vi "Main.vi"() -> ()   [LabVIEW 2020]
panel:
  out "Homogenization Process":u8(slide) scale=0.0..100.0
  out "Internet Connections":string
  out "Raw Material Prices (MYR)":string[][](array[string])
  out "Event Logging":string[][](array[string])
  in  "C\nSell Stock: 3":dbl min=0.0 max=600.0 step=1.0
  in  "Sell Button C":bool
  in  "B\nSell Stock: 2":dbl=1.0 min=0.0 max=932.0 step=1.0
  in  "Sell Button B":bool
  in  "A\nSell Stock:":dbl=1.0 min=0.0 max=950.0 step=1.0
  in  "Sell Button A":bool
  out "Station C\nExport:":dbl
  out "Station B\nStores::":dbl
  out "Station A\nWarehouse:":dbl
  out "Waiting/Running Task:":string caption="Executing Task:"
  out "Time":string
  out "Pipe 13":u8(slide) scale=0.0..100.0
  out "Pipe 12":u8(slide) scale=0.0..100.0
  out "Pipe 11":u8(slide) scale=0.0..100.0
  out "Fragrances":dbl(slide) scale=0.0..100.0
  out "Presevatives":dbl(slide) scale=0.0..100.0
  out "Temperature":dbl[unit](slide) scale=0.0..100.0
  out "Spinning Speed\n       (RPM)":dbl(knob) scale=0.0..20.0
  out "Mixing and Cooling\n          Final Product":dbl(slide) scale=0.0..100.0
  out "Temperature of (B)":dbl[unit](slide) scale=0.0..100.0
  out "(A)+(B)2":u8(slide) scale=0.0..100.0
  out "Spinning Speed\n       (RPM)":dbl(knob) scale=0.0..20.0
  out "Part (B)\nMixing and Heating":dbl(slide) scale=0.0..100.0
  out "Spinning Speed\n      (RPM)":dbl(knob) scale=0.0..20.0
  in  "START":bool
  out "Temperature of \nRaw Material (B)":dbl[unit](slide) scale=0.0..100.0
  out "Main Pipe (B)":u8(slide) scale=0.0..100.0
  out "Main Pipe (B) 2":u8(slide) scale=0.0..100.0
  out "Xanthan Gum\n(w/w)":dbl(slide) scale=0.0..5.0
  out "Pipe 10":u8(slide) scale=0.0..50.0
  out "Glycerol\n(w/w)":dbl(slide) scale=0.0..50.0
  out "Pipe 9":u8(slide) scale=0.0..100.0
  out "Deionized Water\n(w/w)":dbl(slide) scale=0.0..100.0
  out "Pipe 8":u8(slide) scale=0.0..100.0
  out "Temperature of (A)":dbl[unit](slide) scale=0.0..100.0
  out "Temperature of \nRaw Material (A)":dbl[unit](slide) scale=0.0..100.0
  out "(A)+(B)":u8(slide) scale=0.0..100.0
  out "Main Pipe (A)2":u8(slide) scale=0.0..100.0
  out "Part (A)\nMixing and Heating":dbl(slide) scale=0.0..100.0
  out "PEG-40\n(w/w)":dbl(slide) scale=0.0..50.0
  out "Pipe 7":u8(slide) scale=0.0..100.0
  out "Glyceryl Monostearate\n(w/w)":dbl(slide) scale=0.0..50.0
  out "Pipe 6":u8(slide) scale=0.0..100.0
  out "Isopropyl Palmitate\n(w/w)":dbl(slide) scale=0.0..50.0
  out "Pipe 5":u8(slide) scale=0.0..100.0
  out "Mineral Oil\n(w/w)":dbl(slide) scale=0.0..50.0
  out "Pipe 4":u8(slide) scale=0.0..100.0
  out "Pipe 3":u8(slide) scale=0.0..100.0
  out "Petrolatum USP \n(w/w)":dbl(slide) scale=0.0..50.0
  out "Pipe 2":u8(slide) scale=0.0..100.0
  out "Pipe 1":u8(slide) scale=0.0..100.0
  out "Main Pipe (A)":u8(slide) scale=0.0..100.0
  out "Cetyl Alcohol \n(w/w)":dbl(slide) scale=0.0..50.0
  in  "Station to deliver":u16(ring) items=["", "A (Warehouse)", "B (Stores)", "C (Export)"]
  out "Stearic Acid \n(w/w)":dbl(slide) scale=0.0..50.0
  in  "Numbers of Bottles":u16(ring) items=["0", "100", "200", "300", "400", "500"]
  # "Lotion Manufacturing"
  # "100 Bottles per process"
  # "Part (C)\nAdditives"
  # "Deliver to Stations"
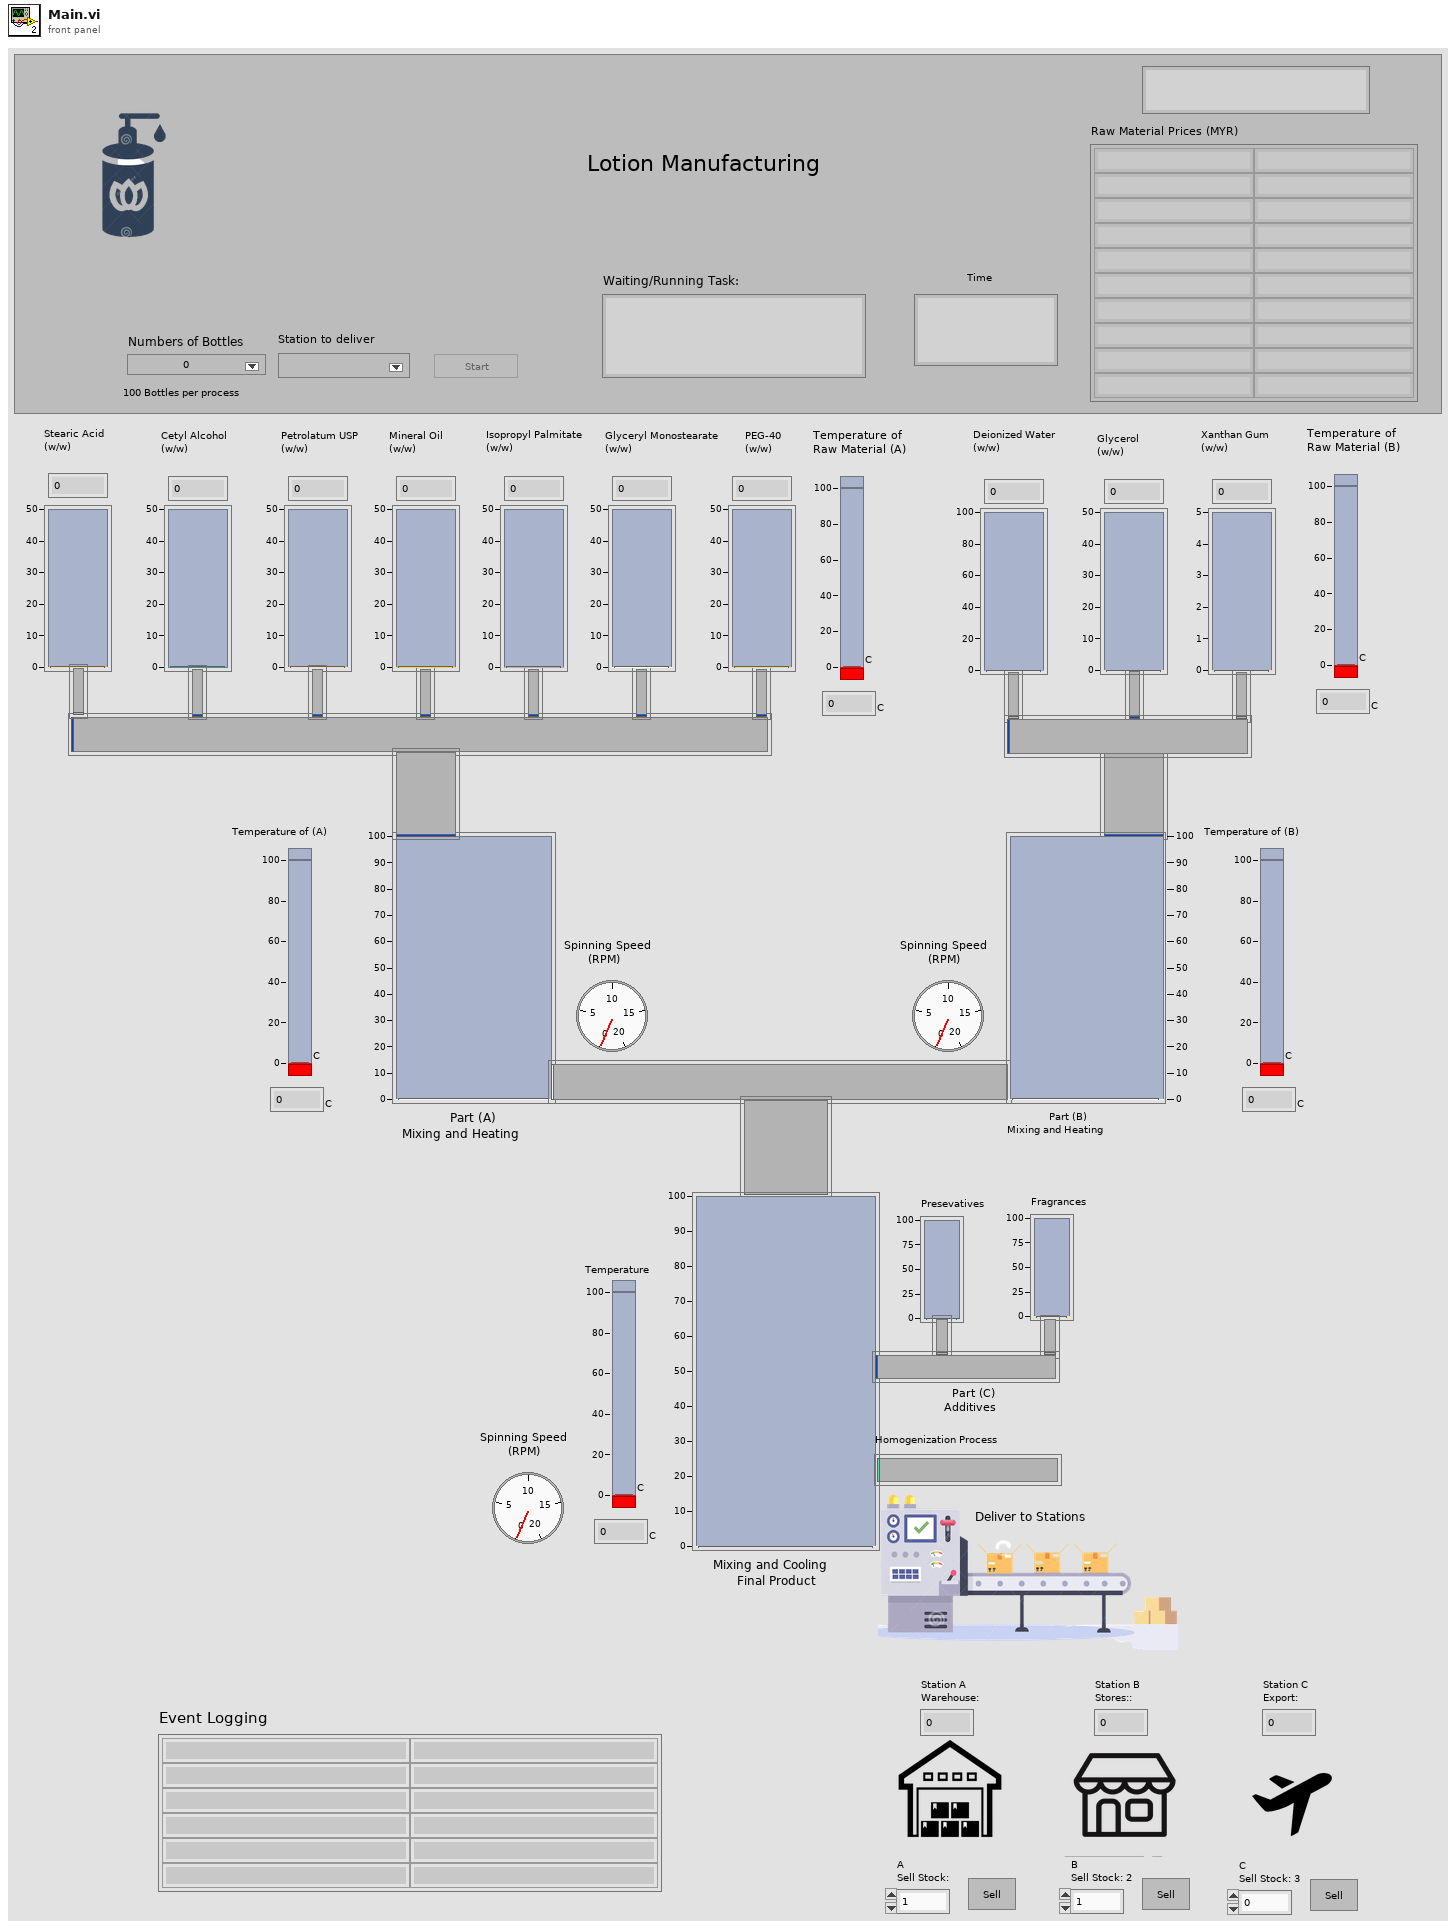
[diagram p1: front panel]
types:
  T1 = enum8{"Enabled", "Disabled", "Disabled and Grayed Out"}
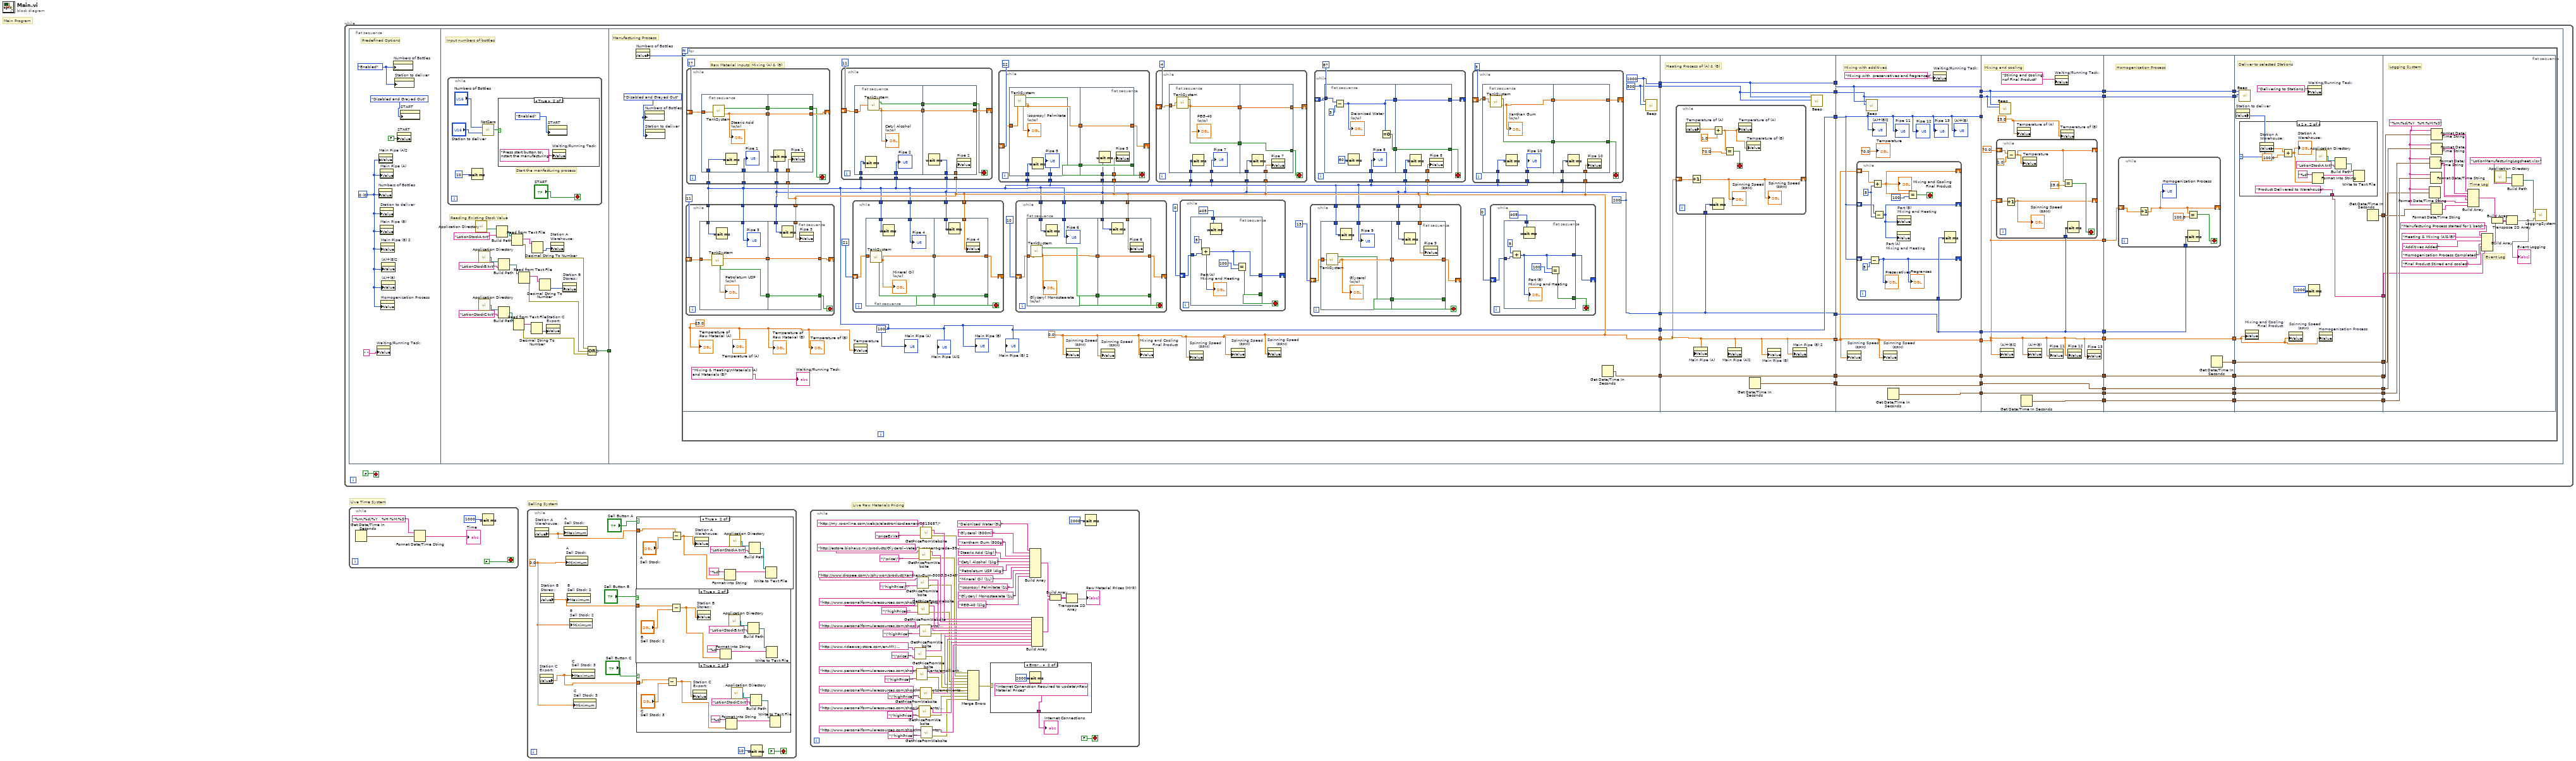
[diagram p0: block diagram]
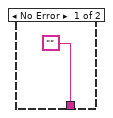
[diagram p2: hidden frame]
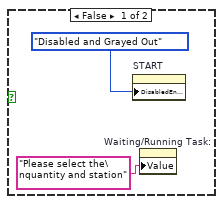
[diagram p6: hidden frame]
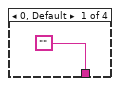
[diagram p7: hidden frame]
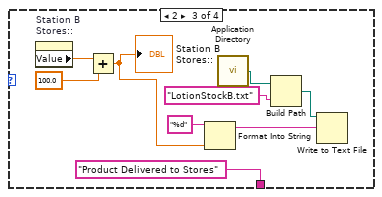
[diagram p8: hidden frame]
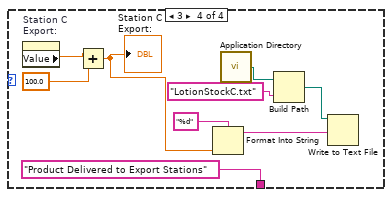
[diagram p9: hidden frame]
diagram:
  # "Live Raw Materials Pricing"
  # "Selling System"
  # "Main Program"
  # "Live Time System"
  n1 = while {
    stop <- FALSE stop-if-true
    n2 = flat-sequence {
      tunnel: [w17] -> w1
      tunnel: w1 -> [_]
      frame #0 {
        w7 = T1."Enabled" ("Disabled")
        w3 = u16 0 items=["0", "100", "200", "300", "400", "500"] ("Numbers of Batch")
        # "Predefined Options"
        n3 = property on="Waiting/Running Task:" class="Str"("Value"=" " ("Executing Task:")) -> ()  [unwired: 2 in, 2 out]
        n4 = property on="Numbers of Bottles" class="Ring (strict)"("Value"=w3) -> ()  [unwired: 2 in, 2 out]
        n5 = property on="Main Pipe (A)2" class="Slide (strict)"("Value"=w3) -> ()  [unwired: 2 in, 2 out]
        n6 = property on="Main Pipe (A)" class="Slide (strict)"("Value"=w3) -> ()  [unwired: 2 in, 2 out]
        n7 = property on="Station to deliver" class="Ring (strict)"("Value"=w3) -> ()  [unwired: 2 in, 2 out]
        n8 = property on="Main Pipe (B)" class="Slide (strict)"("Value"=w3) -> ()  [unwired: 2 in, 2 out]
        n9 = property on="Main Pipe (B) 2" class="Slide (strict)"("Value"=w3) -> ()  [unwired: 2 in, 2 out]
        n10 = property on="Homogenization Process" class="Slide (strict)"("Value"=w3) -> ()  [unwired: 2 in, 2 out]
        n11 = property on="(A)+(B)2" class="Slide (strict)"("Value"=w3) -> ()  [unwired: 2 in, 2 out]
        n12 = property on="(A)+(B)" class="Slide (strict)"("Value"=w3) -> ()  [unwired: 2 in, 2 out]
        n13 = property on="Numbers of Bottles" class="Ring (strict)"("DisabledEnum"=w7) -> ()  [unwired: 2 in, 2 out]
        n14 = property on="Station to deliver" class="Ring (strict)"("DisabledEnum"=w7) -> ()  [unwired: 2 in, 2 out]
        n15 = property on="START" class="Bool (strict)"("Value"=FALSE ("Start/Stop")) -> ()  [unwired: 2 in, 2 out]
        n16 = property on="START" class="Bool (strict)"("DisabledEnum"=T1."Disabled and Grayed Out" ("Disabled")) -> ()  [unwired: 2 in, 2 out]
      }
      frame #1 {
        # "Reading Existing Stock Value"
        # "Input numbers of bottles"
        n17 = while {
          stop <- "START" stop-if-true
          # "Start the manfacturing process"
          n18 = Wait (ms)(milliseconds to wait=u32 10 ("millisecond timer value")) -> ()  [unwired: 1 out]
          n19 = call "NotZero.vi"("Station to deliver"="Station to deliver", "Numbers of Bottles"="Numbers of Bottles") -> ("True"=w27:bool)
          n20 = case shown="True" w27 {
            frame False {
              n21 = property on="START" class="Bool (strict)"("DisabledEnum"=T1."Disabled and Grayed Out" ("Disabled")) -> ()  [unwired: 2 in, 2 out]
              n22 = property on="Waiting/Running Task:" class="Str"("Value"="Please select the\nquantity and station" ("Waiting/Running Task:")) -> ()  [unwired: 2 in, 2 out]
            }
            frame True {
              n23 = property on="START" class="Bool (strict)"("DisabledEnum"=T1."Enabled" ("Disabled")) -> ()  [unwired: 2 in, 2 out]
              n24 = property on="Waiting/Running Task:" class="Str"("Value"="Press start button to\nstart the manufacturing" ("Waiting/Running Task:")) -> ()  [unwired: 2 in, 2 out]
            }
          }
        }
        n25 = call <vilib>:"Application Directory.vi"() -> ("Application Directory"=w16:path)
        n26 = call <vilib>:"Application Directory.vi"() -> ("Application Directory"=w13:path)
        n27 = call <vilib>:"Application Directory.vi"() -> ("Application Directory"=w10:path)
        n28 = Build Path(base path=w16, name or relative path="LotionStockA.txt") -> (appended path=w14:path)
        n29 = Build Path(base path=w13, name or relative path="LotionStockB.txt") -> (appended path=w11:path)
        n30 = Build Path(base path=w10, name or relative path="LotionStockC.txt") -> (appended path=w8:path)
        n31 = Read from Text File(file (use dialog)=w14) -> (text=w23:string, error out=w26:errorcluster)  [unwired: 3 in, 2 out]
        n32 = Read from Text File(file (use dialog)=w8) -> (text=w20:string, error out=w25:errorcluster)  [unwired: 3 in, 2 out]
        n33 = Read from Text File(file (use dialog)=w11) -> (text=w22:string, error out=w18:errorcluster)  [unwired: 3 in, 2 out]
        n34 = Decimal String To Number(string=w20) -> (number=w19:i32)  [unwired: 2 in, 1 out]
        n35 = Decimal String To Number(string=w23) -> (number=w24:i32)  [unwired: 2 in, 1 out]
        n36 = Decimal String To Number(string=w22) -> (number=w21:i32)  [unwired: 2 in, 1 out]
        n37 = property on="Station C\nExport:" class="DigNum (strict)"("Value"=w19) -> ()  [unwired: 2 in, 2 out]
        n38 = property on="Station A\nWarehouse:" class="DigNum (strict)"("Value"=w24) -> ()  [unwired: 2 in, 2 out]
        n39 = property on="Station B\nStores::" class="DigNum (strict)"("Value"=w21) -> ()  [unwired: 2 in, 2 out]
        n40 = Compound Arithmetic op=OR(w26, w18, w25) -> (invert w17:bool)
      }
      frame #2 {
        w36 = T1."Disabled and Grayed Out" ("Disabled")
        # "Manufacturing Process"
        n41 = property on="Numbers of Bottles" class="Ring (strict)"() -> ("Value"=w37:u16)  [unwired: 2 in, 2 out]
        n42 = property on="Numbers of Bottles" class="Ring (strict)"("DisabledEnum"=w36) -> ()  [unwired: 2 in, 2 out]
        n43 = property on="Station to deliver" class="Ring (strict)"("DisabledEnum"=w36) -> ()  [unwired: 2 in, 2 out]
        n44 = for {
          N: w37 -> [_]
          n45 = flat-sequence {
            tunnel: [w89] -> w78
            tunnel: [w88] -> w77
            tunnel: [w87] -> w75
            tunnel: [w86] -> w66
            tunnel: [w84] -> w58
            tunnel: [w85] -> w57
            tunnel: [w303] -> w82
            tunnel: [w308] -> w81
            tunnel: w78 -> [w303]
            tunnel: w77 -> [w309]
            tunnel: [w309] -> w76
            tunnel: w75 -> [w308]
            tunnel: [w307] -> w69
            tunnel: [w306] -> w67
            tunnel: w66 -> [w306]
            tunnel: [w305] -> w62
            tunnel: [w304] -> w61
            tunnel: w58 -> [w304]
            tunnel: w57 -> [w305]
            tunnel: w82 -> [w318]
            tunnel: w81 -> [w327]
            tunnel: [w327] -> w80
            tunnel: [w318] -> w79
            tunnel: w76 -> [w319]
            tunnel: [w324] -> w73
            tunnel: [w323] -> w70
            tunnel: w69 -> [w323]
            tunnel: [w322] -> w68
            tunnel: w67 -> [w322]
            tunnel: w62 -> [w321]
            tunnel: w61 -> [w320]
            tunnel: [w321] -> w60
            tunnel: [w320] -> w59
            tunnel: [w319] -> w40
            tunnel: w80 -> [w340]
            tunnel: w79 -> [w339]
            tunnel: [w339] -> w56
            tunnel: [w346] -> w54
            tunnel: [w345] -> w52
            tunnel: w73 -> [w345]
            tunnel: [w344] -> w50
            tunnel: w70 -> [w344]
            tunnel: [w343] -> w48
            tunnel: w68 -> [w343]
            tunnel: w60 -> [w342]
            tunnel: w59 -> [w341]
            tunnel: [w342] -> w46
            tunnel: [w341] -> w44
            tunnel: [w339] -> w42
            tunnel: [w340] -> w41
            tunnel: w40 -> [_]
            tunnel: w56 -> [w367]
            tunnel: [w367] -> w55
            tunnel: w54 -> [w366]
            tunnel: [w366] -> w53
            tunnel: w52 -> [w365]
            tunnel: [w365] -> w51
            tunnel: w50 -> [w364]
            tunnel: [w364] -> w49
            tunnel: w48 -> [w363]
            tunnel: [w363] -> w47
            tunnel: w46 -> [w362]
            tunnel: [w362] -> w45
            tunnel: w44 -> [w361]
            tunnel: [w361] -> w43
            tunnel: w42 -> [w360]
            tunnel: w41 -> [w359]
            tunnel: [w358] -> w38
            tunnel: w55 -> [w373]
            tunnel: [w382] -> w74
            tunnel: w53 -> [w382]
            tunnel: w51 -> [w381]
            tunnel: [w381] -> w72
            tunnel: [w380] -> w71
            tunnel: w49 -> [w380]
            tunnel: w47 -> [w379]
            tunnel: [w379] -> w65
            tunnel: [w378] -> w64
            tunnel: [w377] -> w63
            tunnel: w45 -> [w376]
            tunnel: w43 -> [w375]
            tunnel: [w374] -> w39
            tunnel: w38 -> [w374]
            tunnel: w74 -> [w437]
            tunnel: w72 -> [w438]
            tunnel: w71 -> [w439]
            tunnel: w65 -> [w430]
            tunnel: w64 -> [w436]
            tunnel: w63 -> [w418]
            tunnel: w39 -> [w431]
            frame #0 {
              w84 = u32 500 ("duration (msec)")
              w85 = u32 1000 ("frequency (Hz)")
              w87 = 200
              w89 = 0.0 ("Spinning Speed")
              w90 = dbl[unit] 25.0 ("Temperature of \nRaw Material (A)")
              w88 = u8 100 ("Slide")
              # "Mixing (A) & (B)"
              # "Raw Material Inputs"
              n46 = while {
                shift-right: [w250] -> _
                shift-left: 11 -> [w257]
                tunnel: w88 -> [w256]
                tunnel: w88 -> [w255]
                tunnel: w87 -> [w254]
                tunnel: w89 -> [w253]
                stop <- w251 stop-if-true
                n47 = flat-sequence {
                  tunnel: w257 -> [w260]
                  tunnel: w256 -> [w262]
                  tunnel: w255 -> [w261]
                  tunnel: [w259] -> w252
                  tunnel: [w258] -> w249
                  tunnel: w254 -> [w266]
                  tunnel: w253 -> [w265]
                  tunnel: [w264] -> w251
                  tunnel: w252 -> [w264]
                  tunnel: [w263] -> w250
                  tunnel: w249 -> [w263]
                  frame #0 {
                    n48 = call "TankSystem.vi"("Input"=w260) -> ("Output"=w259:bool, "Tank"=w258:dbl)
                    "Petrolatum USP \n(w/w)" <- w258
                    n49 = Wait (ms)(milliseconds to wait=w261) -> ()  [unwired: 1 out]
                    "Pipe 3" <- w262
                  }
                  frame #1 {
                    n50 = Wait (ms)(milliseconds to wait=w266) -> ()  [unwired: 1 out]
                    n51 = property on="Pipe 3" class="Slide (strict)"("Value"=w265) -> ()  [unwired: 2 in, 2 out]
                  }
                }
              }
              n52 = while {
                shift-right: [w288] -> _
                shift-left: 27 -> [w293]
                tunnel: w88 -> [w292]
                tunnel: w88 -> [w291]
                tunnel: w87 -> [w290]
                tunnel: w89 -> [w289]
                stop <- w285 stop-if-true
                n53 = flat-sequence {
                  tunnel: w293 -> [w296]
                  tunnel: w292 -> [w298]
                  tunnel: w291 -> [w297]
                  tunnel: [w295] -> w287
                  tunnel: [w294] -> w286
                  tunnel: w290 -> [w302]
                  tunnel: w289 -> [w301]
                  tunnel: [w300] -> w288
                  tunnel: w287 -> [w300]
                  tunnel: w286 -> [w299]
                  tunnel: [w299] -> w285
                  frame #0 {
                    n54 = call "TankSystem.vi"("Input"=w296) -> ("Output"=w294:bool, "Tank"=w295:dbl)
                    "Stearic Acid \n(w/w)" <- w295
                    n55 = Wait (ms)(milliseconds to wait=w298) -> ()  [unwired: 1 out]
                    "Pipe 1" <- w297
                  }
                  frame #1 {
                    n56 = Wait (ms)(milliseconds to wait=w302) -> ()  [unwired: 1 out]
                    n57 = property on="Pipe 1" class="Slide (strict)"("Value"=w301) -> ()  [unwired: 2 in, 2 out]
                  }
                }
              }
              n58 = while {
                shift-right: [w270] -> _
                shift-left: 11 -> [w275]
                tunnel: w88 -> [w274]
                tunnel: w88 -> [w273]
                tunnel: w87 -> [w272]
                tunnel: w89 -> [w271]
                stop <- w267 stop-if-true
                n59 = flat-sequence {
                  tunnel: w275 -> [w278]
                  tunnel: w274 -> [w280]
                  tunnel: w273 -> [w279]
                  tunnel: [w277] -> w269
                  tunnel: [w276] -> w268
                  tunnel: w272 -> [w284]
                  tunnel: w271 -> [w283]
                  tunnel: [w282] -> w270
                  tunnel: w269 -> [w282]
                  tunnel: w268 -> [w281]
                  tunnel: [w281] -> w267
                  frame #0 {
                    n60 = Wait (ms)(milliseconds to wait=w280) -> ()  [unwired: 1 out]
                    n61 = call "TankSystem.vi"("Input"=w278) -> ("Output"=w276:bool, "Tank"=w277:dbl)
                    "Cetyl Alcohol \n(w/w)" <- w277
                    "Pipe 2" <- w279
                  }
                  frame #1 {
                    n62 = Wait (ms)(milliseconds to wait=w284) -> ()  [unwired: 1 out]
                    n63 = property on="Pipe 2" class="Slide (strict)"("Value"=w283) -> ()  [unwired: 2 in, 2 out]
                  }
                }
              }
              n64 = while {
                shift-right: [w239] -> _
                shift-left: 21 -> [w235]
                tunnel: w88 -> [w234]
                tunnel: w88 -> [w233]
                tunnel: w87 -> [w232]
                tunnel: w89 -> [w231]
                stop <- w238 stop-if-true
                n65 = flat-sequence {
                  tunnel: w235 -> [w242]
                  tunnel: [w240] -> w237
                  tunnel: [w241] -> w236
                  tunnel: w234 -> [w244]
                  tunnel: w233 -> [w243]
                  tunnel: [w247] -> w238
                  tunnel: [w248] -> w239
                  tunnel: w237 -> [w248]
                  tunnel: w236 -> [w247]
                  tunnel: w232 -> [w246]
                  tunnel: w231 -> [w245]
                  frame #0 {
                    n66 = call "TankSystem.vi"("Input"=w242) -> ("Output"=w241:bool, "Tank"=w240:dbl)
                    "Mineral Oil\n(w/w)" <- w240
                    n67 = Wait (ms)(milliseconds to wait=w244) -> ()  [unwired: 1 out]
                    "Pipe 4" <- w243
                  }
                  frame #1 {
                    n68 = Wait (ms)(milliseconds to wait=w246) -> ()  [unwired: 1 out]
                    n69 = property on="Pipe 4" class="Slide (strict)"("Value"=w245) -> ()  [unwired: 2 in, 2 out]
                  }
                }
              }
              n70 = property on="Temperature" class="Slide (strict)"("Value"=w90) -> ()  [unwired: 2 in, 2 out]
              n71 = while {
                shift-right: [w221] -> _
                shift-left: 22 -> [w217]
                tunnel: w88 -> [w216]
                tunnel: w88 -> [w215]
                tunnel: w87 -> [w214]
                tunnel: w89 -> [w213]
                stop <- w220 stop-if-true
                n72 = flat-sequence {
                  tunnel: w217 -> [w222]
                  tunnel: [w224] -> w219
                  tunnel: [w223] -> w218
                  tunnel: w216 -> [w226]
                  tunnel: w215 -> [w225]
                  tunnel: [w229] -> w220
                  tunnel: [w230] -> w221
                  tunnel: w219 -> [w230]
                  tunnel: w218 -> [w229]
                  tunnel: w214 -> [w228]
                  tunnel: w213 -> [w227]
                  frame #0 {
                    n73 = call "TankSystem.vi"("Input"=w222) -> ("Output"=w223:bool, "Tank"=w224:dbl)
                    "Isopropyl Palmitate\n(w/w)" <- w224
                    n74 = Wait (ms)(milliseconds to wait=w226) -> ()  [unwired: 1 out]
                    "Pipe 5" <- w225
                  }
                  frame #1 {
                    n75 = Wait (ms)(milliseconds to wait=w228) -> ()  [unwired: 1 out]
                    n76 = property on="Pipe 5" class="Slide (strict)"("Value"=w227) -> ()  [unwired: 2 in, 2 out]
                  }
                }
              }
              n77 = while {
                shift-right: [w203] -> _
                shift-left: 10 -> [w199]
                tunnel: w88 -> [w198]
                tunnel: w88 -> [w197]
                tunnel: w87 -> [w196]
                tunnel: w89 -> [w195]
                stop <- w202 stop-if-true
                n78 = flat-sequence {
                  tunnel: w199 -> [w204]
                  tunnel: [w205] -> w201
                  tunnel: [w206] -> w200
                  tunnel: w198 -> [w208]
                  tunnel: w197 -> [w207]
                  tunnel: [w211] -> w202
                  tunnel: [w212] -> w203
                  tunnel: w201 -> [w212]
                  tunnel: w200 -> [w211]
                  tunnel: w196 -> [w210]
                  tunnel: w195 -> [w209]
                  frame #0 {
                    n79 = call "TankSystem.vi"("Input"=w204) -> ("Output"=w206:bool, "Tank"=w205:dbl)
                    "Glyceryl Monostearate\n(w/w)" <- w205
                    n80 = Wait (ms)(milliseconds to wait=w208) -> ()  [unwired: 1 out]
                    "Pipe 6" <- w207
                  }
                  frame #1 {
                    n81 = Wait (ms)(milliseconds to wait=w210) -> ()  [unwired: 1 out]
                    n82 = property on="Pipe 6" class="Slide (strict)"("Value"=w209) -> ()  [unwired: 2 in, 2 out]
                  }
                }
              }
              n83 = property on="Spinning Speed\n       (RPM)" class="Knob (strict)"("Value"=w89) -> ()  [unwired: 2 in, 2 out]
              n84 = property on="Spinning Speed\n      (RPM)" class="Knob (strict)"("Value"=w89) -> ()  [unwired: 2 in, 2 out]
              n85 = property on="Mixing and Cooling\n          Final Product" class="Slide (strict)"("Value"=w89) -> ()  [unwired: 2 in, 2 out]
              n86 = while {
                shift-right: [w177] -> _
                shift-left: 4 -> [w185]
                tunnel: w88 -> [w184]
                tunnel: w88 -> [w183]
                tunnel: w87 -> [w182]
                tunnel: w89 -> [w181]
                stop <- w179 stop-if-true
                n87 = flat-sequence {
                  tunnel: w185 -> [w186]
                  tunnel: w184 -> [w190]
                  tunnel: w183 -> [w189]
                  tunnel: [w188] -> w180
                  tunnel: [w187] -> w178
                  tunnel: w182 -> [w194]
                  tunnel: w181 -> [w193]
                  tunnel: w180 -> [w192]
                  tunnel: [w192] -> w179
                  tunnel: w178 -> [w191]
                  tunnel: [w191] -> w177
                  frame #0 {
                    n88 = call "TankSystem.vi"("Input"=w186) -> ("Output"=w188:bool, "Tank"=w187:dbl)
                    "PEG-40\n(w/w)" <- w187
                    n89 = Wait (ms)(milliseconds to wait=w190) -> ()  [unwired: 1 out]
                    "Pipe 7" <- w189
                  }
                  frame #1 {
                    n90 = Wait (ms)(milliseconds to wait=w194) -> ()  [unwired: 1 out]
                    n91 = property on="Pipe 7" class="Slide (strict)"("Value"=w193) -> ()  [unwired: 2 in, 2 out]
                  }
                }
              }
              n92 = while {
                shift-right: [w167] -> _
                shift-left: 0 -> [w168]
                stop <- w170 stop-if-true
                n93 = flat-sequence {
                  tunnel: w168 -> [w175]
                  tunnel: u32 405 ("millisecond timer value") -> [w176]
                  tunnel: [w171] -> w170
                  tunnel: [w172] -> w167
                  frame #0 {
                    n94 = Add(x=5, y=w175) -> (x+y=w172:i32)
                    "Part (A)\nMixing and Heating" <- w172
                    n95 = Wait (ms)(milliseconds to wait=w176) -> ()  [unwired: 1 out]
                    n96 = Equal?(x=w172, y=100) -> (x = y?=w171:bool)
                  }
                }
              }
              n97 = property on="Spinning Speed\n       (RPM)" class="Knob (strict)"("Value"=w89) -> ()  [unwired: 2 in, 2 out]
              n98 = property on="Spinning Speed\n      (RPM)" class="Knob (strict)"("Value"=w89) -> ()  [unwired: 2 in, 2 out]
              n99 = property on="Spinning Speed\n       (RPM)" class="Knob (strict)"("Value"=w89) -> ()  [unwired: 2 in, 2 out]
              n100 = while {
                shift-right: [w139] -> _
                shift-left: 13 -> [w135]
                tunnel: w88 -> [w134]
                tunnel: w88 -> [w133]
                tunnel: w87 -> [w132]
                tunnel: w89 -> [w131]
                stop <- w138 stop-if-true
                n101 = flat-sequence {
                  tunnel: w135 -> [w142]
                  tunnel: [w141] -> w137
                  tunnel: [w140] -> w136
                  tunnel: w134 -> [w144]
                  tunnel: w133 -> [w143]
                  tunnel: [w147] -> w138
                  tunnel: [w148] -> w139
                  tunnel: w137 -> [w148]
                  tunnel: w136 -> [w147]
                  tunnel: w132 -> [w146]
                  tunnel: w131 -> [w145]
                  frame #0 {
                    n102 = call "TankSystem.vi"("Input"=w142) -> ("Output"=w140:bool, "Tank"=w141:dbl)
                    "Glycerol\n(w/w)" <- w141
                    n103 = Wait (ms)(milliseconds to wait=w144) -> ()  [unwired: 1 out]
                    "Pipe 9" <- w143
                  }
                  frame #1 {
                    n104 = Wait (ms)(milliseconds to wait=w146) -> ()  [unwired: 1 out]
                    n105 = property on="Pipe 9" class="Slide (strict)"("Value"=w145) -> ()  [unwired: 2 in, 2 out]
                  }
                }
              }
              n106 = while {
                shift-right: [w152] -> _
                shift-left: 87 -> [w155]
                tunnel: w88 -> [w151]
                tunnel: w89 -> [w150]
                tunnel: w87 -> [w149]
                stop <- w154 stop-if-true
                n107 = flat-sequence {
                  tunnel: w155 -> [w161]
                  tunnel: [w162] -> w156
                  tunnel: [w159] -> w153
                  tunnel: w151 -> [w158]
                  tunnel: [w166] -> w154
                  tunnel: w156 -> [w166]
                  tunnel: w153 -> [w165]
                  tunnel: [w165] -> w152
                  tunnel: w150 -> [w164]
                  tunnel: w149 -> [w163]
                  frame #0 {
                    n108 = Subtract(x=w161, y=3) -> (x-y=w159:i32)
                    "Deionized Water\n(w/w)" <- w159
                    n109 = Wait (ms)(milliseconds to wait=u32 80) -> ()  [unwired: 1 out]
                    n110 = Equal To 0?(x=w159) -> (x = 0?=w162:bool)
                    "Pipe 8" <- w158
                  }
                  frame #1 {
                    n111 = Wait (ms)(milliseconds to wait=w163) -> ()  [unwired: 1 out]
                    n112 = property on="Pipe 8" class="Slide (strict)"("Value"=w164) -> ()  [unwired: 2 in, 2 out]
                  }
                }
              }
              n113 = while {
                shift-right: [w117] -> _
                shift-left: 3 -> [w120]
                tunnel: w88 -> [w116]
                tunnel: w88 -> [w115]
                tunnel: w87 -> [w114]
                tunnel: w89 -> [w113]
                stop <- w119 stop-if-true
                n114 = flat-sequence {
                  tunnel: w120 -> [w124]
                  tunnel: [w123] -> w121
                  tunnel: [w122] -> w118
                  tunnel: w116 -> [w126]
                  tunnel: w115 -> [w125]
                  tunnel: [w130] -> w119
                  tunnel: w121 -> [w130]
                  tunnel: w118 -> [w129]
                  tunnel: [w129] -> w117
                  tunnel: w114 -> [w128]
                  tunnel: w113 -> [w127]
                  frame #0 {
                    n115 = call "TankSystem.vi"("Input"=w124) -> ("Output"=w123:bool, "Tank"=w122:dbl)
                    "Xanthan Gum\n(w/w)" <- w122
                    n116 = Wait (ms)(milliseconds to wait=w126) -> ()  [unwired: 1 out]
                    "Pipe 10" <- w125
                  }
                  frame #1 {
                    n117 = Wait (ms)(milliseconds to wait=w128) -> ()  [unwired: 1 out]
                    n118 = property on="Pipe 10" class="Slide (strict)"("Value"=w127) -> ()  [unwired: 2 in, 2 out]
                  }
                }
              }
              n119 = while {
                shift-right: [w103] -> _
                shift-left: 0 -> [w104]
                stop <- w106 stop-if-true
                n120 = flat-sequence {
                  tunnel: w104 -> [w109]
                  tunnel: u32 405 ("millisecond timer value") -> [w112]
                  tunnel: [w110] -> w106
                  tunnel: [w107] -> w103
                  frame #0 {
                    n121 = Add(x=5, y=w109) -> (x+y=w107:i32)
                    "Part (B)\nMixing and Heating" <- w107
                    n122 = Wait (ms)(milliseconds to wait=w112) -> ()  [unwired: 1 out]
                    n123 = Equal?(x=w107, y=100) -> (x = y?=w110:bool)
                  }
                }
              }
              n124 = Get Date/Time In Seconds() -> (seconds since 1Jan1904=w86:timestamp)
              n125 = call <vilib>:"Beep.vi"("duration (msec)"=w84, "frequency (Hz)"=w85) -> ()  [unwired: 10 in]
              "Main Pipe (A)" <- w88
              "Main Pipe (A)2" <- w88
              "Temperature of \nRaw Material (A)" <- w90
              "Temperature of (A)" <- w90
              "Main Pipe (B) 2" <- w88
              "Main Pipe (B)" <- w88
              "Temperature of \nRaw Material (B)" <- w90
              "Temperature of (B)" <- w90
              "Waiting/Running Task:" <- "Mixing & Heating\nMaterials (A) and Materials (B)" ("Executing Task:")
            }
            frame #1 {
              # "Heating Process of (A) & (B)"
              n126 = while {
                shift-right: [w311] -> _
                shift-left: w303 -> [w310]
                tunnel: w308 -> [w312]
                stop <- w314 stop-if-true
                n127 = property on="Temperature of (A)" class="Slide (strict)"() -> ("Value"=w316:dbl[unit])  [unwired: 2 in, 2 out]
                n128 = Increment(x=w310) -> (x+1=w311:dbl)
                "Spinning Speed\n       (RPM)" <- w311
                "Spinning Speed\n      (RPM)" <- w311
                n129 = Wait (ms)(milliseconds to wait=w312) -> ()  [unwired: 1 out]
                n130 = Add(x=w316, y=dbl[unit] 1.0) -> (x+y=w313:dbl[unit])
                n131 = Equal?(x=w313, y=dbl[unit] 70.0) -> (x = y?=w314:bool)
                n132 = property on="Temperature of (A)" class="Slide (strict)"("Value"=w313) -> ()  [unwired: 2 in, 2 out]
                n133 = property on="Temperature of (B)" class="Slide (strict)"("Value"=w313) -> ()  [unwired: 2 in, 2 out]
              }
              n134 = property on="Main Pipe (A)" class="Slide (strict)"("Value"=w303) -> ()  [unwired: 2 in, 2 out]
              n135 = property on="Main Pipe (A)2" class="Slide (strict)"("Value"=w303) -> ()  [unwired: 2 in, 2 out]
              n136 = Get Date/Time In Seconds() -> (seconds since 1Jan1904=w307:timestamp)
              n137 = property on="Main Pipe (B)" class="Slide (strict)"("Value"=w303) -> ()  [unwired: 2 in, 2 out]
              n138 = property on="Main Pipe (B) 2" class="Slide (strict)"("Value"=w303) -> ()  [unwired: 2 in, 2 out]
              n139 = call <vilib>:"Beep.vi"("duration (msec)"=w304, "frequency (Hz)"=w305) -> ()  [unwired: 10 in]
            }
            frame #2 {
              # "Mixing with additives"
              n140 = property on="Spinning Speed\n      (RPM)" class="Knob (strict)"("Value"=w318) -> ()  [unwired: 2 in, 2 out]
              n141 = while {
                shift-right: [w335] -> _
                shift-left: w318 -> [w338]
                shift-right: [w332] -> _
                shift-left: w319 -> [w333]
                tunnel: w327 -> [w331]
                shift-right: [w328] -> _
                shift-left: w319 -> [w330]
                stop <- w336 stop-if-true
                w334 = 5 ("y")
                n142 = Subtract(x=w330, y=u8 5) -> (x-y=w328:u8)
                "Fragrances" <- w328
                "Presevatives" <- w328
                n143 = Add(x=w338, y=w334) -> (x+y=w335:dbl)
                "Mixing and Cooling\n          Final Product" <- w335
                n144 = Subtract(x=w333, y=w334) -> (x-y=w332:i32)
                n145 = property on="Part (A)\nMixing and Heating" class="Slide (strict)"("Value"=w332) -> ()  [unwired: 2 in, 2 out]
                n146 = property on="Part (B)\nMixing and Heating" class="Slide (strict)"("Value"=w332) -> ()  [unwired: 2 in, 2 out]
                n147 = Equal?(x=w335, y=100) -> (x = y?=w336:bool)
                n148 = Wait (ms)(milliseconds to wait=w331) -> ()  [unwired: 1 out]
              }
              n149 = call <vilib>:"Beep.vi"("duration (msec)"=w320, "frequency (Hz)"=w321) -> ()  [unwired: 10 in]
              n150 = property on="Spinning Speed\n       (RPM)" class="Knob (strict)"("Value"=w318) -> ()  [unwired: 2 in, 2 out]
              n151 = Get Date/Time In Seconds() -> (seconds since 1Jan1904=w324:timestamp)
              n152 = property on="Waiting/Running Task:" class="Str"("Value"="Mixing with  preservatives and fragrances" ("Executing Task:")) -> ()  [unwired: 2 in, 2 out]
              "(A)+(B)" <- w319
              "(A)+(B)2" <- w319
              "Temperature" <- dbl[unit] 70.0 ("Temperature")
              "Pipe 11" <- w319
              "Pipe 12" <- w319
              "Pipe 13" <- w319
            }
            frame #3 {
              w347 = dbl[unit] 25.0 ("Temperature of (A)")
              # "Mixing and cooling"
              n153 = while {
                shift-right: [w355] -> _
                shift-left: dbl[unit] 70.0 ("Temperature") -> [w357]
                shift-right: [w351] -> _
                shift-left: w339 -> [w352]
                tunnel: w340 -> [w350]
                stop <- w353 stop-if-true
                n154 = Increment(x=w352) -> (x+1=w351:dbl)
                "Spinning Speed\n       (RPM)" <- w351
                n155 = Subtract(x=w357, y=dbl[unit] 1.0) -> (x-y=w355:dbl[unit])
                n156 = property on="Temperature" class="Slide (strict)"("Value"=w355) -> ()  [unwired: 2 in, 2 out]
                n157 = Equal?(x=w355, y=dbl[unit] 25.0) -> (x = y?=w353:bool)
                n158 = Wait (ms)(milliseconds to wait=w350) -> ()  [unwired: 1 out]
              }
              n159 = call <vilib>:"Beep.vi"("duration (msec)"=w341, "frequency (Hz)"=w342) -> ()  [unwired: 10 in]
              n160 = property on="(A)+(B)2" class="Slide (strict)"("Value"=w339) -> ()  [unwired: 2 in, 2 out]
              n161 = property on="Temperature of (A)" class="Slide (strict)"("Value"=w347) -> ()  [unwired: 2 in, 2 out]
              n162 = Get Date/Time In Seconds() -> (seconds since 1Jan1904=w346:timestamp)
              n163 = property on="(A)+(B)" class="Slide (strict)"("Value"=w339) -> ()  [unwired: 2 in, 2 out]
              n164 = property on="Pipe 11" class="Slide (strict)"("Value"=w339) -> ()  [unwired: 2 in, 2 out]
              n165 = property on="Waiting/Running Task:" class="Str"("Value"="Stirring and cooling\nof Final Product" ("Executing Task:")) -> ()  [unwired: 2 in, 2 out]
              n166 = property on="Temperature of (B)" class="Slide (strict)"("Value"=w347) -> ()  [unwired: 2 in, 2 out]
              n167 = property on="Pipe 12" class="Slide (strict)"("Value"=w339) -> ()  [unwired: 2 in, 2 out]
              n168 = property on="Pipe 13" class="Slide (strict)"("Value"=w339) -> ()  [unwired: 2 in, 2 out]
            }
            frame #4 {
              # "Homogenization Process"
              n169 = while {
                shift-right: [w369] -> _
                shift-left: w360 -> [w372]
                tunnel: w359 -> [w370]
                stop <- w368 stop-if-true
                n170 = Increment(x=w372) -> (x+1=w369:dbl)
                "Homogenization Process" <- w369
                n171 = Equal?(x=w369, y=100.0) -> (x = y?=w368:bool)
                n172 = Wait (ms)(milliseconds to wait=w370) -> ()  [unwired: 1 out]
              }
              n173 = Get Date/Time In Seconds() -> (seconds since 1Jan1904=w358:timestamp)
            }
            frame #5 {
              # "Deliver to selected Stations"
              n174 = property on="Station to deliver" class="Ring (strict)"() -> ("Value"=w384:u16)  [unwired: 2 in, 2 out]
              n175 = call <vilib>:"Beep.vi"("duration (msec)"=w375, "frequency (Hz)"=w376) -> ()  [unwired: 10 in]
              n176 = case shown="1" w384 {
                tunnel: ["" "Product Delivered to Warehouse" "Product Delivered to Stores" "Product Delivered to Export Stations"] -> w377
                frame 0, Default {
                }
                frame 1 {
                  n177 = property on="Station A\nWarehouse:" class="DigNum (strict)"() -> ("Value"=w395:dbl)  [unwired: 2 in, 2 out]
                  n178 = Add(x=w395, y=100.0) -> (x+y=w392:dbl)
                  "Station A\nWarehouse:" <- w392
                  n179 = Format Into String(format string="%d", w392) -> (resulting string=w393:string)  [unwired: 2 in, 1 out]
                  n180 = call <vilib>:"Application Directory.vi"() -> ("Application Directory"=w389:path)
                  n181 = Build Path(base path=w389, name or relative path="LotionStockA.txt") -> (appended path=w387:path)
                  n182 = Write to Text File(file (use dialog)=w387, text=w393) -> ()  [unwired: 2 in, 3 out]
                }
                frame 2 {
                  n183 = property on="Station B\nStores::" class="DigNum (strict)"() -> ("Value"=w404:dbl)  [unwired: 2 in, 2 out]
                  n184 = Add(x=w404, y=100.0) -> (x+y=w401:dbl)
                  "Station B\nStores::" <- w401
                  n185 = Format Into String(format string="%d", w401) -> (resulting string=w402:string)  [unwired: 2 in, 1 out]
                  n186 = call <vilib>:"Application Directory.vi"() -> ("Application Directory"=w398:path)
                  n187 = Build Path(base path=w398, name or relative path="LotionStockB.txt") -> (appended path=w396:path)
                  n188 = Write to Text File(file (use dialog)=w396, text=w402) -> ()  [unwired: 2 in, 3 out]
                }
                frame 3 {
                  n189 = property on="Station C\nExport:" class="DigNum (strict)"() -> ("Value"=w413:dbl)  [unwired: 2 in, 2 out]
                  n190 = Add(x=w413, y=100.0) -> (x+y=w410:dbl)
                  "Station C\nExport:" <- w410
                  n191 = Format Into String(format string="%d", w410) -> (resulting string=w411:string)  [unwired: 2 in, 1 out]
                  n192 = call <vilib>:"Application Directory.vi"() -> ("Application Directory"=w407:path)
                  n193 = Build Path(base path=w407, name or relative path="LotionStockC.txt") -> (appended path=w405:path)
                  n194 = Write to Text File(file (use dialog)=w405, text=w411) -> ()  [unwired: 2 in, 3 out]
                }
              }
              n195 = property on="Mixing and Cooling\n          Final Product" class="Slide (strict)"("Value"=w373) -> ()  [unwired: 2 in, 2 out]
              n196 = property on="Spinning Speed\n       (RPM)" class="Knob (strict)"("Value"=w373) -> ()  [unwired: 2 in, 2 out]
              n197 = property on="Waiting/Running Task:" class="Str"("Value"="Delivering to Stations..." ("Executing Task:")) -> ()  [unwired: 2 in, 2 out]
              n198 = Wait (ms)(milliseconds to wait=u32 1000 ("millisecond timer value")) -> ()  [unwired: 1 out]
              n199 = property on="Homogenization Process" class="Slide (strict)"("Value"=w373) -> ()  [unwired: 2 in, 2 out]
              n200 = Get Date/Time In Seconds() -> (seconds since 1Jan1904=w378:timestamp)
            }
            frame #6 {
              w432 = "%m/%d/%Y  %H:%M:%S" ("time format string (%c)")
              # "Logging System"
              # "Event Log"
              # "Time Log"
              n201 = Format Date/Time String(time format string (%c)=w432, seconds (now)=w431) -> (date/time string=w425:string)  [unwired: 1 in]
              n202 = Format Date/Time String(time format string (%c)=w432, seconds (now)=w438) -> (date/time string=w427:string)  [unwired: 1 in]
              n203 = Format Date/Time String(time format string (%c)=w432, seconds (now)=w437) -> (date/time string=w426:string)  [unwired: 1 in]
              n204 = Format Date/Time String(time format string (%c)=w432, seconds (now)=w430) -> (date/time string=w429:string)  [unwired: 1 in]
              n205 = Format Date/Time String(time format string (%c)=w432, seconds (now)=w439) -> (date/time string=w428:string)  [unwired: 1 in]
              n206 = Format Date/Time String(time format string (%c)=w432, seconds (now)=w436) -> (date/time string=w424:string)  [unwired: 1 in]
              n207 = Build Array(w429, w428, w427, w426, w425, w424) -> (w416:string[])
              n208 = Build Array("Manufacturing Process started for 1 batch", "Heating & Mixing (A)&(B)", "Additives Added", "Homogenization Process Completed", "Final Product Stirred and cooled", w418) -> (w417:string[])
              n209 = Build Array(w416, w417) -> (w415:string[][])
              n210 = call <vilib>:"Application Directory.vi"() -> ("Application Directory"=w434:path)
              n211 = Transpose 2D Array(2D array=w415) -> (transposed array=w414:string[][])
              "Event Logging" <- w414
              n212 = Build Path(base path=w434, name or relative path="LotionManufacturingLogsheet.xlsx") -> (appended path=w433:path)
              n213 = call "LoggingSystem.vi"("Array"=w414, "Path"=w433) -> ()
            }
          }
        }
      }
    }
  }
  n214 = while {
    stop <- FALSE stop-if-true
    n215 = Get Date/Time In Seconds() -> (seconds since 1Jan1904=w444:timestamp)
    n216 = Format Date/Time String(time format string (%c)="%m/%d/%Y   %H:%M:%S", seconds (now)=w444) -> (date/time string=→"Time":string)  [unwired: 1 in]
    n217 = Wait (ms)(milliseconds to wait=u32 1000 ("millisecond timer value")) -> ()  [unwired: 1 out]
  }
  n218 = while {
    stop <- FALSE stop-if-true
    w445 = 0.0 ("Data Entry Limits:Minimum")
    n219 = property on="Station A\nWarehouse:" class="DigNum (strict)"() -> ("Value"=w452:dbl)  [unwired: 2 in, 2 out]
    n220 = property on="Station C\nExport:" class="DigNum (strict)"() -> ("Value"=w446:dbl)  [unwired: 2 in, 2 out]
    n221 = property on="Station B\nStores::" class="DigNum (strict)"() -> ("Value"=w451:dbl)  [unwired: 2 in, 2 out]
    n222 = property on="A\nSell Stock:" class="DigNum (strict)"("Maximum"=w452) -> ()  [unwired: 2 in, 2 out]
    n223 = property on="A\nSell Stock:" class="DigNum (strict)"("Minimum"=w445) -> ()  [unwired: 2 in, 2 out]
    n224 = property on="B\nSell Stock: 2" class="DigNum (strict)"("Maximum"=w451) -> ()  [unwired: 2 in, 2 out]
    n225 = property on="B\nSell Stock: 2" class="DigNum (strict)"("Minimum"=w445) -> ()  [unwired: 2 in, 2 out]
    n226 = property on="C\nSell Stock: 3" class="DigNum (strict)"("Maximum"=w446) -> ()  [unwired: 2 in, 2 out]
    n227 = property on="C\nSell Stock: 3" class="DigNum (strict)"("Minimum"=w445) -> ()  [unwired: 2 in, 2 out]
    n228 = case shown="True" "Sell Button B" {
      tunnel: w451 -> [_ w469]
      frame False {
      }
      frame True {
        n229 = Subtract(x=w469, y="B\nSell Stock: 2") -> (x-y=w466:dbl)
        n230 = property on="Station B\nStores::" class="DigNum (strict)"("Value"=w466) -> ()  [unwired: 2 in, 2 out]
        n231 = Format Into String(format string="%d", w466) -> (resulting string=w467:string)  [unwired: 2 in, 1 out]
        n232 = call <vilib>:"Application Directory.vi"() -> ("Application Directory"=w464:path)
        n233 = Build Path(base path=w464, name or relative path="LotionStockB.txt") -> (appended path=w462:path)
        n234 = Write to Text File(file (use dialog)=w462, text=w467) -> ()  [unwired: 2 in, 3 out]
      }
    }
    n235 = case shown="True" "Sell Button A" {
      tunnel: w452 -> [_ w477]
      frame False {
      }
      frame True {
        n236 = Subtract(x=w477, y="A\nSell Stock:") -> (x-y=w474:dbl)
        n237 = property on="Station A\nWarehouse:" class="DigNum (strict)"("Value"=w474) -> ()  [unwired: 2 in, 2 out]
        n238 = Format Into String(format string="%d", w474) -> (resulting string=w475:string)  [unwired: 2 in, 1 out]
        n239 = call <vilib>:"Application Directory.vi"() -> ("Application Directory"=w472:path)
        n240 = Build Path(base path=w472, name or relative path="LotionStockA.txt") -> (appended path=w470:path)
        n241 = Write to Text File(file (use dialog)=w470, text=w475) -> ()  [unwired: 2 in, 3 out]
      }
    }
    n242 = case shown="True" "Sell Button C" {
      tunnel: w446 -> [_ w461]
      frame False {
      }
      frame True {
        n243 = Subtract(x=w461, y="C\nSell Stock: 3") -> (x-y=w458:dbl)
        n244 = property on="Station C\nExport:" class="DigNum (strict)"("Value"=w458) -> ()  [unwired: 2 in, 2 out]
        n245 = Format Into String(format string="%d", w458) -> (resulting string=w459:string)  [unwired: 2 in, 1 out]
        n246 = call <vilib>:"Application Directory.vi"() -> ("Application Directory"=w456:path)
        n247 = Build Path(base path=w456, name or relative path="LotionStockC.txt") -> (appended path=w454:path)
        n248 = Write to Text File(file (use dialog)=w454, text=w459) -> ()  [unwired: 2 in, 3 out]
      }
    }
    n249 = Wait (ms)(milliseconds to wait=u32 10 ("millisecond timer value")) -> ()  [unwired: 1 out]
  }
  n250 = while {
    stop <- FALSE ("status") stop-if-true
    n251 = call "GetPriceFromWebsite.vi"("Search String"="\"price\"", "Website In"="http://www.rideawaystore.com/en-MY/Battles-White-Petroleum-Jelly-Skin-Supplement/r50206397.htm?colour=White&sku=1188824&productid=317771&gclid=Cj0KCQjws4aKBhDPARIsAIWH0JUVJucQvzTj3tvCGOhznq3I_Wv_KhDtTwWSn6CFNTMeipATPFHXcCMaAqjbEALw_wcB") -> ("error out"=w485:errorcluster, "Result Price"=w503:string)  [unwired: 1 in, 1 out]
    n252 = call "GetPriceFromWebsite.vi"("Search String"="\"highPrice\"", "Website In"="http://www.personalformularesources.com/shop/ingredients/emollients/mineral-oil/") -> ("error out"=w484:errorcluster, "Result Price"=w500:string)  [unwired: 1 in, 1 out]
    n253 = call "GetPriceFromWebsite.vi"("Search String"="\"highPrice\":", "Website In"="http://www.dropee.com/v/phywon/product/Xanthan-Gum-500G/34348") -> ("error out"=w488:errorcluster, "Result Price"=w512:string)  [unwired: 1 in, 1 out]
    n254 = call "GetPriceFromWebsite.vi"("Search String"="\"highPrice\"", "Website In"="http://www.personalformularesources.com/shop/ingredients/emulsifiers-thickeners/stearic-acid/") -> ("error out"=w487:errorcluster, "Result Price"=w506:string)  [unwired: 1 in, 1 out]
    n255 = call "GetPriceFromWebsite.vi"("Search String"="\"price\">" ("search string"), "Website In"="http://estore.biohaus.my/products/Glycerol--Vetec™-reagent-grade--99-/1427") -> ("error out"=w489:errorcluster, "Result Price"=w515:string)  [unwired: 1 in, 1 out]
    n256 = call "GetPriceFromWebsite.vi"("Search String"="\"highPrice\"", "Website In"="http://www.personalformularesources.com/shop/ingredients/emulsifiers-thickeners/additives-glyceryl-monostearate/") -> ("error out"=w482:errorcluster, "Result Price"=w494:string)  [unwired: 1 in, 1 out]
    n257 = call "GetPriceFromWebsite.vi"("Search String"="\"highPrice\"", "Website In"="http://www.personalformularesources.com/shop/ingredients/emulsifiers-thickeners/cetyl-alcohol/") -> ("error out"=w486:errorcluster, "Result Price"=w507:string)  [unwired: 1 in, 1 out]
    n258 = call "GetPriceFromWebsite.vi"("Search String"="\"highPrice\"", "Website In"="http://www.personalformularesources.com/shop/ingredients/emollients/isopropyl-myristate/") -> ("error out"=w483:errorcluster, "Result Price"=w497:string)  [unwired: 1 in, 1 out]
    n259 = call "GetPriceFromWebsite.vi"("Search String"="priceExVat" ("search string"), "Website In"="http://my.rs-online.com/web/p/electronics-cleaners/2513687/" ("URL")) -> ("error out"=w490:errorcluster, "Result Price"=w518:string)  [unwired: 1 in, 1 out]
    n260 = call "GetPriceFromWebsite.vi"("Search String"="\"highPrice\"", "Website In"="http://www.personalformularesources.com/shop/ingredients/emulsifiers-thickeners/peg-40-hydrogenated-castor-oil/") -> ("error out"=w481:errorcluster, "Result Price"=w491:string)  [unwired: 1 in, 1 out]
    n261 = Merge Errors(w490, w489, w488, w487, w486, w485, w484, w483, w482, w481) -> (w479:errorcluster)
    n262 = case shown="Error .." w479 {
      tunnel: ["" "Internet Conenction Required to update\nRaw Material Prices" ("Internet Connections")] -> w478
      frame No Error {
      }
      frame Error {
        n263 = Wait (ms)(milliseconds to wait=u32 2000) -> ()  [unwired: 1 out]
      }
    }
    "Internet Connections" <- w478
    n264 = Build Array("Deionized Water (5L)", "Glycerol (500ml)", "Xantham Gum (500g)", "Stearic Acid (1kg) ", "Cetyl Alcohol (1kg)", "Petrolatum USP (4kg)", "Mineral Oil (1L) ", "Isopropyl Palmitate (1L)", "Glyceryl Monostearate (1L)", "PEG-40 (1kg)") -> (w524:string[])
    n265 = Build Array(w518, w515, w512, w506, w507, w503, w500, w497, w494, w491) -> (w523:string[])
    n266 = Build Array(w524, w523) -> (w522:string[][])
    n267 = Transpose 2D Array(2D array=w522) -> (transposed array=→"Raw Material Prices (MYR)":string[][])
    n268 = Wait (ms)(milliseconds to wait=u32 2000) -> ()  [unwired: 1 out]
  }
